vi "Get Marker Coordinates.vi"(6 "Text":string, 7 "Source VI":refnum<vi>, 8 "Current Coords":T1, 9 "Init Coords":T1, 10 "Type":T3, 11 "Graph Ref":refnum<vi>) -> (2 "Markers":T2, 3 "Cancelled":bool)   [LabVIEW 2019]
uses:
  controls/markerType.ctl
  controls/MarkerInfo.ctl
  <vilib>/Utility/miscctls.llb/LVPoint32TypeDef.ctl
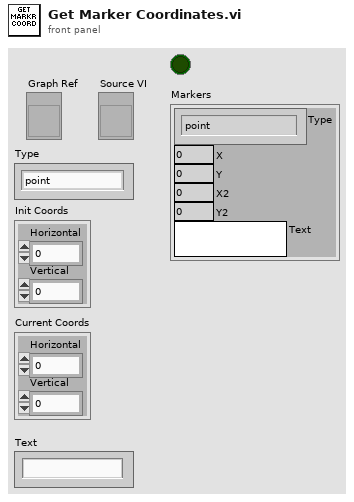
[diagram p1: front panel]
types:
  T1 = typedef "LVPoint32TypeDef.ctl" = cluster{"Horizontal":i32, "Vertical":i32}
  T2 = typedef "MarkerInfo.ctl" = cluster{"Type":T3, "X":dbl, "Y":dbl, "X2":dbl, "Y2":dbl, "Text":string}
  T3 = typedef "markerType.ctl" = enum16{"point", "arrow", "horiz", "vert", "vert range", "horiz range", "box"}
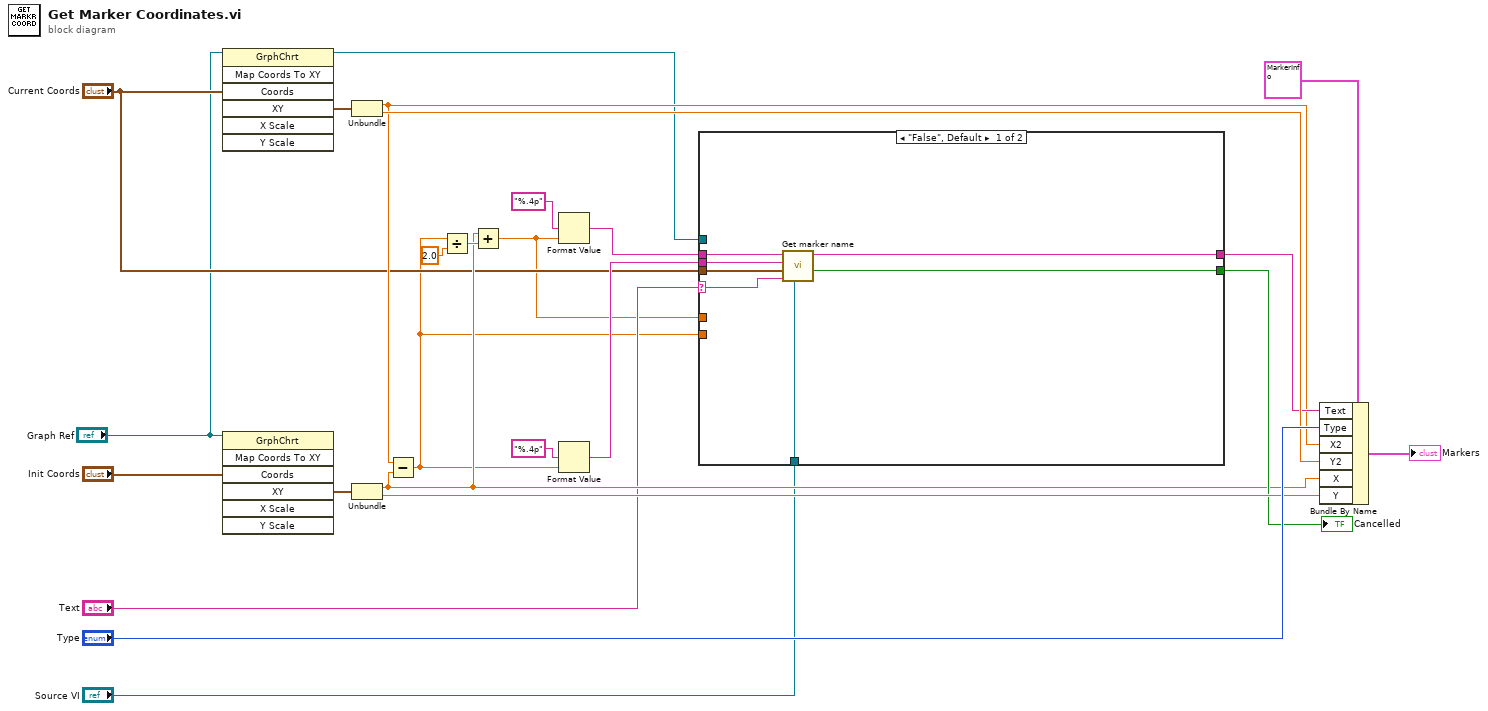
[diagram p0: block diagram]
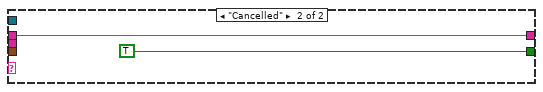
[diagram p2: hidden frame]
diagram:
  n1 = invoke class="GrphChrt" method="Map Coords To XY"(reference="Graph Ref", "Coords"="Current Coords") -> (reference out=w6:refnum<vi>, "XY"=w21:cluster{"X":dbl, "Y":dbl})  [unwired: 5 in, 5 out]
  n2 = invoke class="GrphChrt" method="Map Coords To XY"(reference="Graph Ref", "Coords"="Init Coords") -> ("XY"=w22:cluster{"X":dbl, "Y":dbl})  [unwired: 5 in, 6 out]
  n3 = Unbundle(w21) -> ("X"=w16:dbl, "Y"=w19:dbl)
  n4 = Unbundle(w22) -> ("X"=w9:dbl, "Y"=w20:dbl)
  n5 = Subtract(x=w16, y=w9) -> (x-y=w2:dbl)
  n6 = Divide(x=w2, y=2.0) -> (x/y=w12:dbl)
  n7 = Add(x=w9, y=w12) -> (x+y=w3:dbl)
  n8 = Format Value(format string="%.4p", value (0)=w3) -> (output string=w11:string)  [unwired: 1 in]
  n9 = Format Value(format string="%.4p", value (0)=w2) -> (output string=w10:string)  [unwired: 1 in]
  n10 = case shown="\"False\", Default" "Text" {
    selector: "Text" -> [w27 _]
    tunnel: [w32 w34] -> w18
    tunnel: [w31 TRUE ("cancelled")] -> w17
    tunnel: w11 -> [w30 w34]
    tunnel: w10 -> [w29 _]
    tunnel: "Current Coords" -> [w28 _]
    tunnel: w6 -> [_ _]
    tunnel: "Source VI" -> [w26 _]
    tunnel: w3 -> [_ _]
    tunnel: w2 -> [_ _]
    frame "False", Default {
      n11 = call "Get marker name.vi"("Source VI"=w26, "Text"=w27, "Cursor Pos"=w28, "BW"=w29, "Fc"=w30) -> ("cancelled"=w31:bool, "text"=w32:string)  [unwired: 5 in]
    }
    frame "Cancelled" {
    }
  }
  "Cancelled" <- w17
  n12 = Bundle By Name(cluster=T2 {"Type"=enum."vert", "X"=2.0, "Y"=2.0, "X2"=2.0, "Y2"=2.0, "Text"="Drag and click to\nposition a marker"} ("Markers"), "Text"=w18, "Type"="Type", "X2"=w16, "Y2"=w19, "X"=w9, "Y"=w20) -> (→"Markers":T2)
